vi "Fetch Measurement(Single Point).vi"(0 "VISA resource name":refnum<visa-resource-name>, 11 "error in (no error)":errorcluster) -> (4 "VISA resource name out":refnum<visa-resource-name>, 6 "Measurement":sgl, 15 "error out":errorcluster)   [LabVIEW 2010, in "Agilent 3458.lvlib"]
doc: "Retrieves a single measurement from the output buffer after the sample count has been set in the configure multipoint(set to 1) and the trigger count has been set in the read Measurement(Single Point) which is also set to 1.\n\n<B>Note:</B> Use this VI only with other low-level VIs. The high-level VIs automatically incorporate this functionality. This VI does not check the instrument status. If you want to check the instrument status, call the Error Query VI at the conclusion of the sequence."
uses:
  <instrlib>/Agilent 3458/Agilent 3458.lvlib
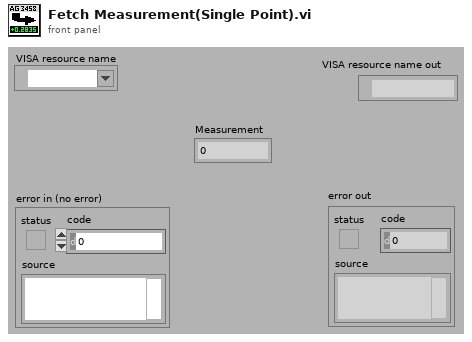
[diagram p1: front panel]
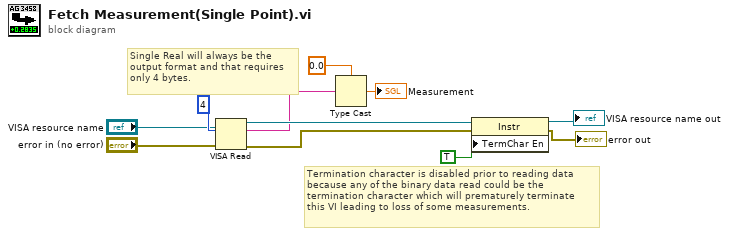
[diagram p0: block diagram]
diagram:
  # "Termination character is disabled prior to reading data\nbecause any of the binary data read could be the \ntermination character which will prematurely terminate\nthis VI leading to loss of some measurements."
  # "Single Real will always be the\noutput format and that requires\nonly 4 bytes."
  n1 = VISA Read(VISA resource name="VISA resource name", byte count=u32 4, error in (no error)="error in (no error)") -> (VISA resource name out=w10:refnum<visa-resource-name>, read buffer=w6:string, error out=w9:errorcluster)  [unwired: 1 out]
  n2 = Type Cast(type=sgl 0.0, x=w6) -> (*(type *) &x=→"Measurement":sgl)
  n3 = property class="Instr"(reference=w10, error in=w9, "TermChar En"=TRUE) -> (reference out=→"VISA resource name out":refnum<visa-resource-name>, error out=→"error out":errorcluster)
